vi "Calculate miniscan pixels XY only.vi"(8 "No of Z planes":i32=1, 9 "Resolution multiplier":dbl=1.0, 10 "XY Coordinates (zero based)":i32[](array[numeric])) -> (1 "Number of lines":dbl, 3 "Pixels in ROI":dbl, 4 "X pixels":dbl)   [LabVIEW 2020]
panel:
  out "error out":errorcluster
  in  "error in":errorcluster
  in  "Z Step":dbl=1.0
  # "Pixels in miniscan"
  # "X start\nY start\nX stop\nY stop"
  # "Z Start\nZ Stop"
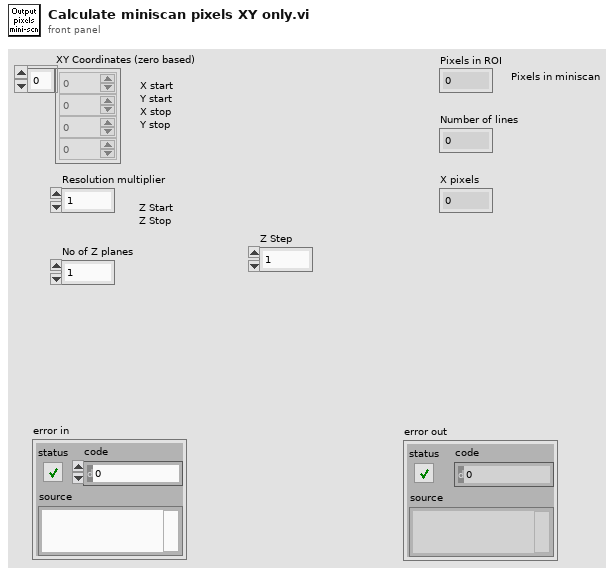
[diagram p1: front panel]
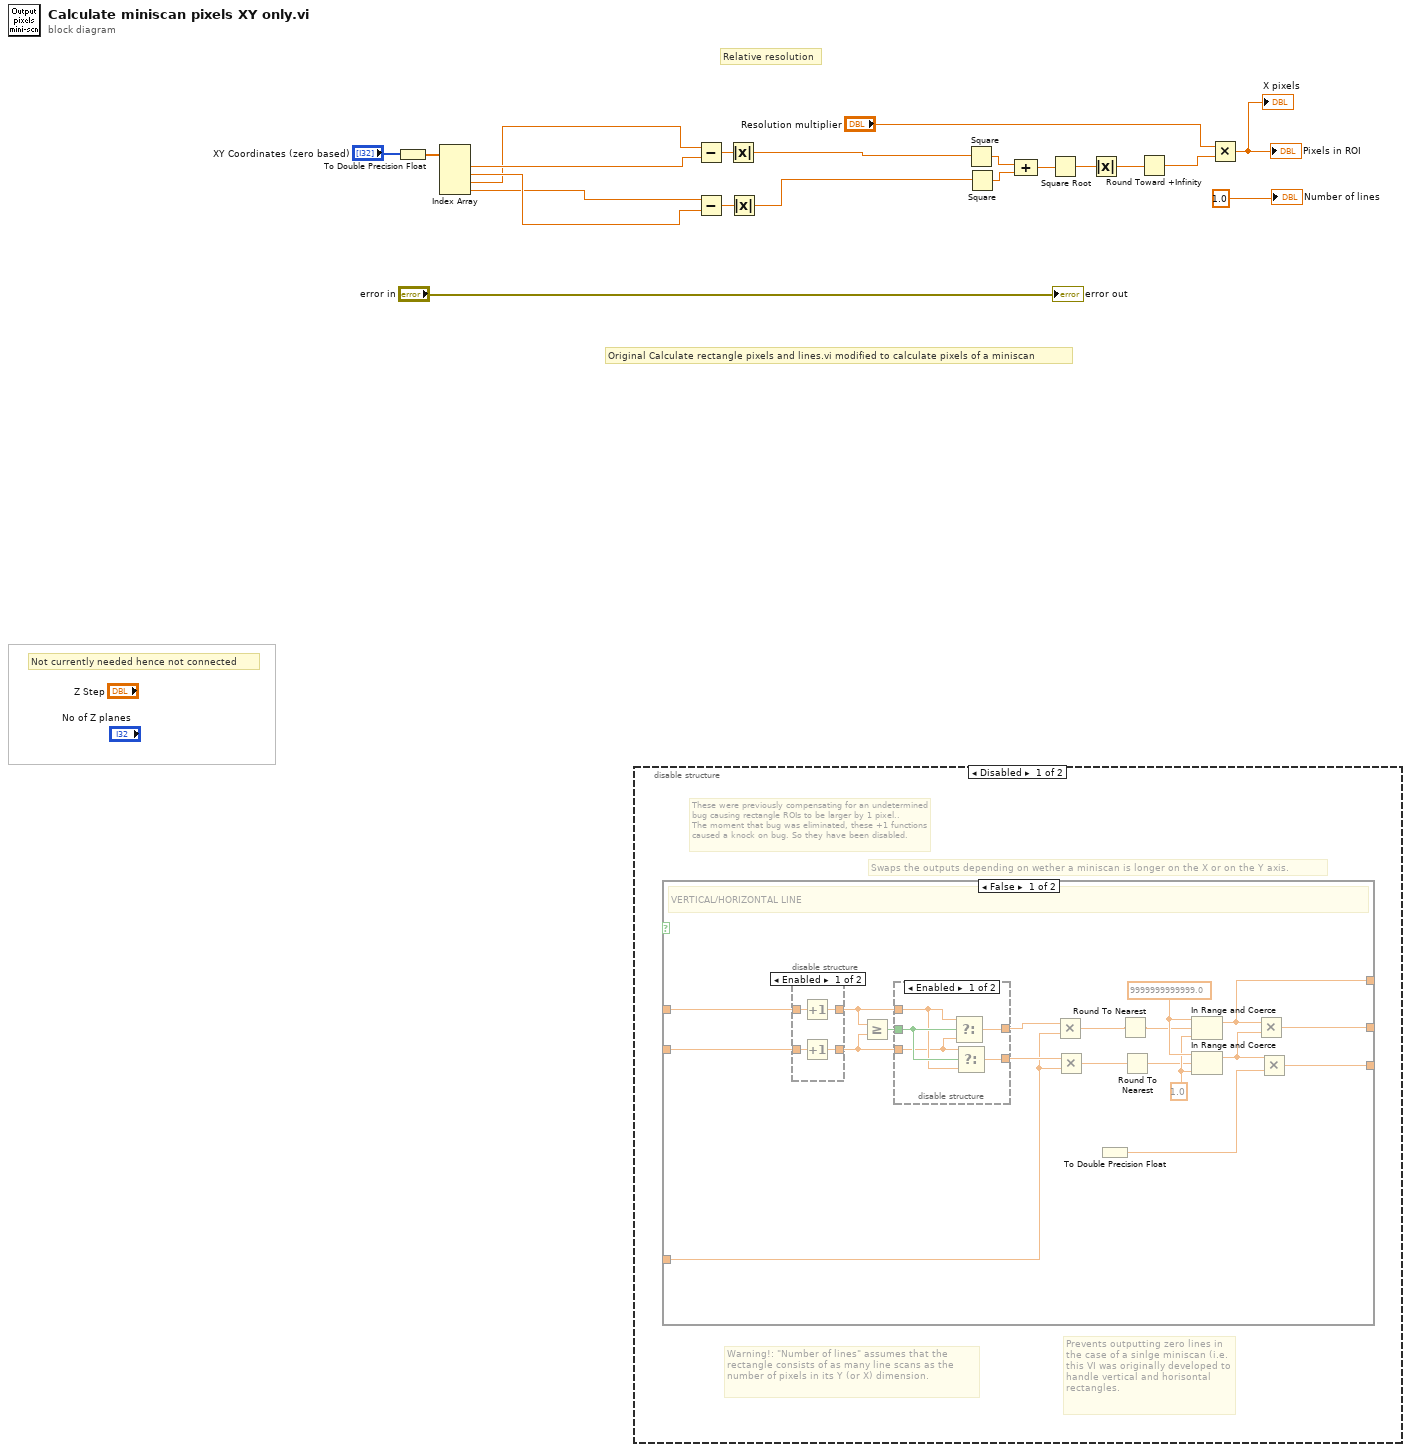
[diagram p0: block diagram]
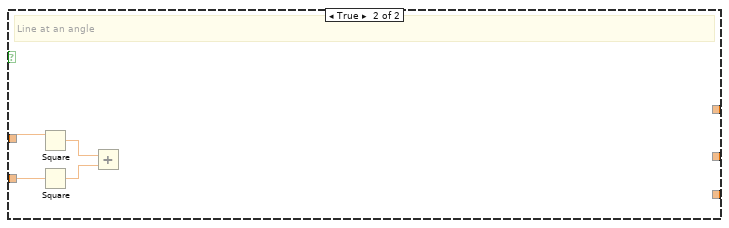
[diagram p4: hidden frame]
diagram:
  # "Original Calculate rectangle pixels and lines.vi modified to calculate pixels of a miniscan"
  # "Not currently needed hence not connected"
  # "Relative resolution"
  n1 = To Double Precision Float(number="XY Coordinates (zero based)") -> (double precision float=w2:dbl[])
  n2 = Index Array(array=w2) -> (element #1=w18:dbl, element #2=w17:dbl, element #3=w16:dbl, element #4=w15:dbl)  [unwired: 4 in]
  n3 = disable-structure shown="Disabled" {
    frame Disabled {
      # "These were previously compensating for an undetermined bug causing rectangle ROIs to be larger by 1 pixel..\nThe moment that bug was eliminated, these +1 functions caused a knock on bug. So they have been disabled."
      # "Prevents outputting zero lines in the case of a sinlge miniscan (i.e. this VI was originally developed to handle vertical and horisontal rectangles."
      # "Warning!: \"Number of lines\" assumes that the rectangle consists of as many line scans as the number of pixels in its Y (or X) dimension."
      # "Swaps the outputs depending on wether a miniscan is longer on the X or on the Y axis."
      n4 = case shown="False" {
        selector: _ -> [_ _]
        tunnel: [w38 _] -> _
        tunnel: [w33 _] -> _
        tunnel: [w30 _] -> _
        tunnel: _ -> [w27 _]
        tunnel: _ -> [w22 w56]
        tunnel: _ -> [w21 w55]
        frame False {
          w36 = 1.0 ("lower limit")
          w37 = 9999999999999.0 ("upper limit")
          # "VERTICAL/HORIZONTAL LINE"
          n5 = disable-structure shown="Enabled" {
            disable-tunnel: w22 -> [w50 w52]
            disable-tunnel: w21 -> [w49 w51]
            disable-tunnel: [w48 w52] -> w35
            disable-tunnel: [w47 w51] -> w34
            frame Enabled {
              n6 = Increment(x=w50) -> (x+1=w48:dbl)
              n7 = Increment(x=w49) -> (x+1=w47:dbl)
            }
            frame Disabled {
            }
          }
          n8 = Greater Or Equal?(x=w35, y=w34) -> (x >= y?=w39:bool)
          n9 = disable-structure shown="Enabled" {
            disable-tunnel: w39 -> [w44 _]
            disable-tunnel: [w43 w46] -> w29
            disable-tunnel: [w42 w45] -> w28
            disable-tunnel: w35 -> [w41 w45]
            disable-tunnel: w34 -> [w40 w46]
            frame Enabled {
              n10 = Select(t=w41, s=w44, f=w40) -> (s? t:f=w43:dbl)
              n11 = Select(t=w40, s=w44, f=w41) -> (s? t:f=w42:dbl)
            }
            frame Disabled {
            }
          }
          n12 = Multiply(x=w29, y=w27) -> (x*y=w26:dbl)
          n13 = Multiply(x=w28, y=w27) -> (x*y=w24:dbl)
          n14 = To Double Precision Float() -> (double precision float=w31:dbl)  [unwired: 1 in]
          n15 = Round To Nearest(number=w26) -> (nearest integer value=w25:dbl)
          n16 = Round To Nearest(number=w24) -> (nearest integer value=w23:dbl)
          n17 = In Range and Coerce(upper limit=w37, x=w25, lower limit=w36) -> (coerced(x)=w38:dbl)  [unwired: 1 out]
          n18 = In Range and Coerce(upper limit=w37, x=w23, lower limit=w36) -> (coerced(x)=w32:dbl)  [unwired: 1 out]
          n19 = Multiply(x=w38, y=w32) -> (x*y=w33:dbl)
          n20 = Multiply(x=w32, y=w31) -> (x*y=w30:dbl)
        }
        frame True {
          # "Line at an angle"
          n21 = Square(x=w56) -> (x^2=w54:dbl)
          n22 = Square(x=w55) -> (x^2=w53:dbl)
          n23 = Add(x=w54, y=w53) -> ()  [unwired: 1 out]
        }
      }
    }
    frame Enabled {
    }
  }
  n24 = Subtract(x=w16, y=w18) -> (x-y=w19:dbl)
  n25 = Subtract(x=w15, y=w17) -> (x-y=w20:dbl)
  n26 = Absolute Value(x=w19) -> (abs(x)=w14:dbl)
  n27 = Absolute Value(x=w20) -> (abs(x)=w13:dbl)
  n28 = Square(x=w14) -> (x^2=w10:dbl)
  n29 = Square(x=w13) -> (x^2=w11:dbl)
  n30 = Compound Arithmetic op=ADD(w10, w11) -> (w9:dbl)
  n31 = Square Root(x=w9) -> (sqrt(x)=w8:dbl)
  n32 = Absolute Value(x=w8) -> (abs(x)=w7:dbl)
  n33 = Round Toward +Infinity(x=w7) -> (ceil(x): smallest int >= x=w6:dbl)
  n34 = Multiply(x="Resolution multiplier", y=w6) -> (x*y=→"Pixels in ROI" →"X pixels":dbl)
  "error out" <- "error in"
  "Number of lines" <- 1.0
